vi "Img_Center_Crop.vi"(8 "error in (no error)":errorcluster, 9 "height":i32, 10 "width":i32, 11 "Image In":T1) -> (0 "error out":errorcluster, 3 "Image Out":T1)   [LabVIEW 2020]
uses:
  <vilib>/vision/Image Controls.llb/IMAQ Image.ctl
  <vilib>/vision/NI_Vision_Development_Module.lvlib
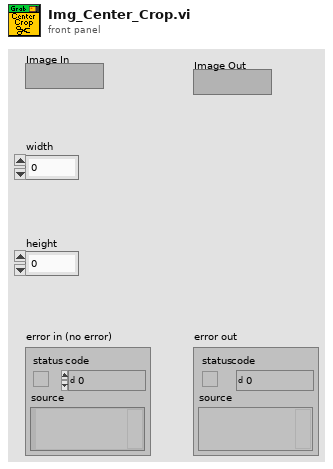
[diagram p1: front panel]
types:
  T1 = typedef "IMAQ Image.ctl" = refnum<image>
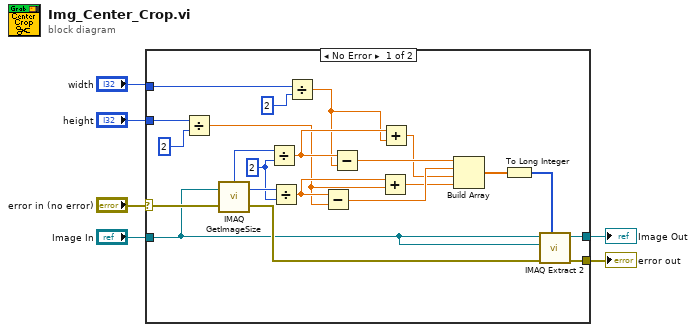
[diagram p0: block diagram]
diagram:
  n1 = case shown="No Error" "error in (no error)" {
    selector: "error in (no error)" -> [w9 w29]
    tunnel: "width" -> [w25 _]
    tunnel: "height" -> [w22 _]
    tunnel: [w12 _] -> w4
    tunnel: "Image In" -> [w8 _]
    tunnel: [w7 w29] -> w1
    frame No Error {
      w26 = 2
      n2 = Divide(x=w22, y=2) -> (x/y=w18:dbl)
      n3 = call "IMAQ GetImageSize"("Image"=w8, "error in (no error)"=w9) -> ("Y Resolution"=w28:i32, "X Resolution"=w27:i32, "error out"=w10:errorcluster)  [unwired: 2 in]
      n4 = Divide(x=w27, y=w26) -> (x/y=w21:dbl)
      n5 = Divide(x=w28, y=w26) -> (x/y=w19:dbl)
      n6 = Divide(x=w25, y=2) -> (x/y=w20:dbl)
      n7 = Subtract(x=w19, y=w18) -> (x-y=w16:dbl)
      n8 = Subtract(x=w21, y=w20) -> (x-y=w17:dbl)
      n9 = Add(x=w19, y=w18) -> (x+y=w14:dbl)
      n10 = Add(x=w21, y=w20) -> (x+y=w15:dbl)
      n11 = Build Array(w17, w16, w15, w14) -> (w13:dbl[])
      n12 = To Long Integer(number=w13) -> (32bit integer=w11:i32[])
      n13 = call "IMAQ Extract 2"("Optional Rectangle"=w11, "error in (no error)"=w10, "Image Dst"=w8, "Image Src"=w8) -> ("error out"=w7:errorcluster, "Image Dst Out"=w12:T1)  [unwired: 6 in]
    }
    frame Error {
    }
  }
  "Image Out" <- w4
  "error out" <- w1
